vi "get_acq_number.vi"(7 "reset acq. number?":bool, 8 "error in (no error)":errorcluster) -> (0 "error out":errorcluster, 1 "# of acq":i32, 2 "# of meas cycles":i32, 3 "VISA resource name out":refnum<visa-resource-name>)   [LabVIEW 2011]
doc: "returns the number of meas cycle calculate based on the number of acq. divided by the number of frames\n\nThe number is only updated after an acquisition and is set to zero after a setting changed. Can be updated by setting the \"reset acq. number\" to true which simply starts a measurement which in turn updates the acq. number. Otherwise it will read the old number and the counting wont be correct..."
uses:
  global.vi
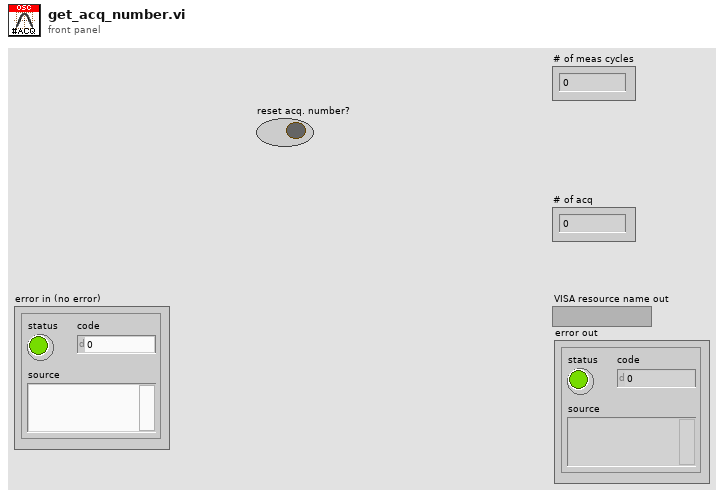
[diagram p1: front panel]
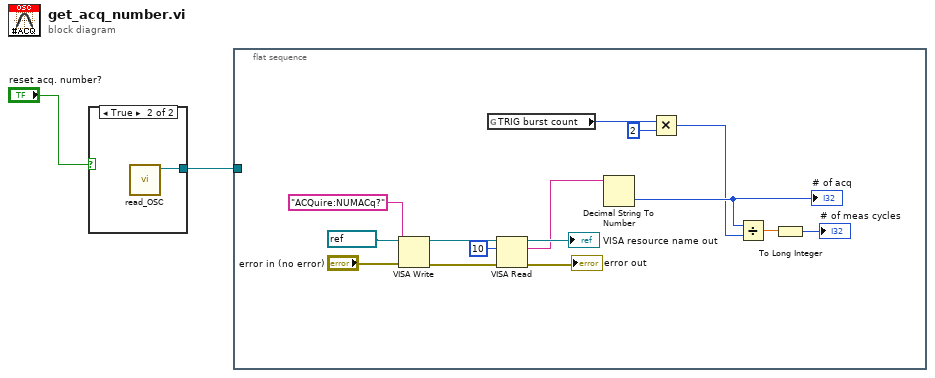
[diagram p0: block diagram]
diagram:
  n1 = case shown="True" "reset acq. number?" {
    tunnel: [_ w3] -> w1
    frame False {
    }
    frame True {
      n2 = call "read_OSC.vi"() -> ("VISA resource name out"=w3:refnum<visa-resource-name>)  [unwired: 8 in, 3 out]
    }
  }
  n3 = flat-sequence {
    tunnel: w1 -> [_]
    frame #0 {
      n4 = VISA Write(VISA resource name=refnum<visa-resource-name> "OSC", write buffer="ACQuire:NUMACq?", error in (no error)="error in (no error)") -> (VISA resource name out=w16:refnum<visa-resource-name>, error out=w12:errorcluster)  [unwired: 1 out]
      n5 = global read "global.vi" "TRIG burst count"() -> (w6:i32)
      n6 = VISA Read(VISA resource name=w16, byte count=u32 10, error in (no error)=w12) -> (VISA resource name out=→"VISA resource name out":refnum<visa-resource-name>, read buffer=w10:string, error out=→"error out":errorcluster)  [unwired: 1 out]
      n7 = Decimal String To Number(string=w10) -> (number=w9:i32)  [unwired: 2 in, 1 out]
      "# of acq" <- w9
      n8 = Multiply(x=w6, y=2) -> (x*y=w4:i32)
      n9 = Divide(x=w9, y=w4) -> (x/y=w8:dbl)
      n10 = To Long Integer(number=w8) -> (32bit integer=→"# of meas cycles":i32)
    }
  }
